vi "Get Size and CRC for new.vi"() -> ()   [LabVIEW 2024]
uses:
  <userlib>/_OpenG.lib/file/file.llb/openg_file.lvlib
panel:
  out "data size":i32
  out "CRC32Value":u32 format="%x"
  out "error out":errorcluster
  in  "error in (no error)":errorcluster
  in  "Working Dir In":path
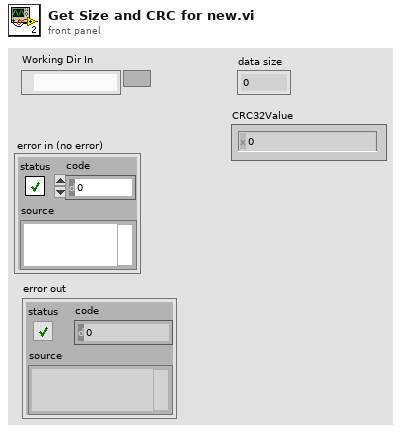
[diagram p1: front panel]
types:
  T1 = typedef "openg_file.lvlib/File Info Record__ogtk.ctl" = cluster{"type":string, "creator":string, "permissions":i32, "data size":i32, "res size":i32, "creation date":u32, "modification date":u32, "bFolder":bool, "bInvisible":bool, "location":cluster{"vertical":i16, "horizontal":i16}, "owner":string, "group":string}
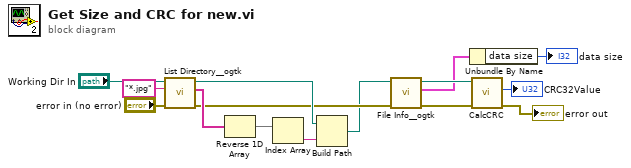
[diagram p0: block diagram]
diagram:
  n1 = call <userlib>:"List Directory__ogtk.vi"("error in (no error)"="error in (no error)", "pattern"="*.jpg", "directory path"="Working Dir In") -> ("error out"=w8:errorcluster, "file names"=w12:string[], "dup directory path"=w11:path)  [unwired: 1 in, 1 out]
  n2 = Reverse 1D Array(array=w12) -> (reversed array=w10:string[])
  n3 = Index Array(array=w10) -> (element=w9:string)  [unwired: 1 in]
  n4 = Build Path(base path=w11, name or relative path=w9) -> (appended path=w7:path)
  n5 = call <userlib>:"File Info__ogtk.vi"("error in (no error)"=w8, "file"=w7) -> ("error out"=w5:errorcluster, "file info"=w2:T1, "file out"=w6:path)  [unwired: 4 in]
  n6 = Unbundle By Name(w2) -> ("data size"=→"data size":i32)
  n7 = call "CalcCRC.vi"("error in (no error)"=w5, "FileToCalculate"=w6) -> ("error out"=→"error out":errorcluster, "CRC32Value"=→"CRC32Value":u32)  [unwired: 7 in, 1 out]
